vi "CostEvaluation.vi"(0 "Packet Size":i32, 1 "Ratio":dbl format="%#_13g", 3 "Channel":T1, 4 "method":enum16{"Edited", "original"}(ring)) -> (5 "delay(s)":dbl)   [LabVIEW 2014]
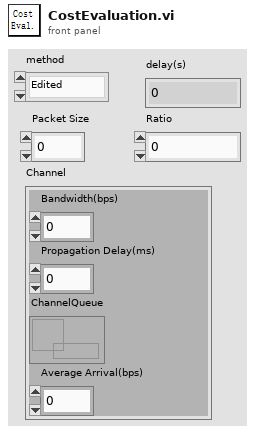
[diagram p1: front panel]
types:
  T1 = cluster{"Bandwidth(bps)":i32, "Propagation Delay(ms)":i32, "ChannelQueue":refnum<queue>, "Average Arrival(bps)":dbl}
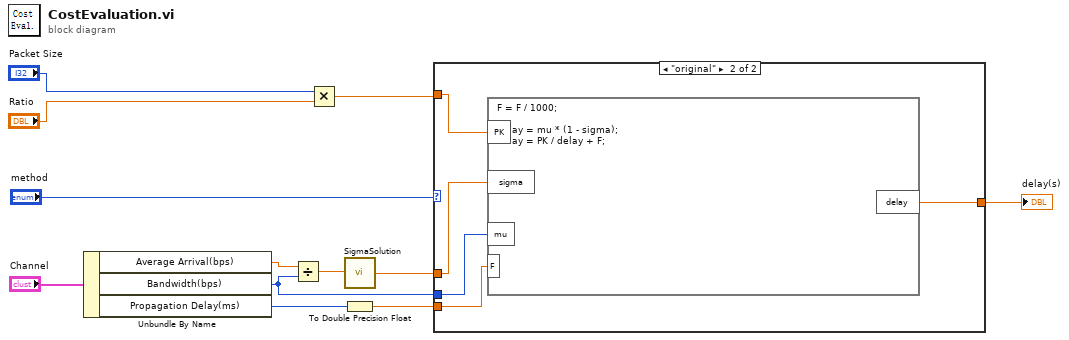
[diagram p0: block diagram]
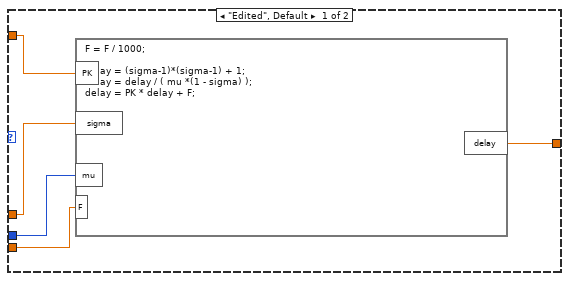
[diagram p2: hidden frame]
diagram:
  n1 = Unbundle By Name("Channel") -> ("Average Arrival(bps)"=w7:dbl, "Bandwidth(bps)"=w3:i32, "Propagation Delay(ms)"=w4:i32)
  n2 = Divide(x=w7, y=w3) -> (x/y=w6:dbl)
  n3 = Multiply(x="Packet Size", y="Ratio") -> (x*y=w9:dbl)
  n4 = call "SigmaSolution.vi"("rou"=w6) -> ("sigma"=w5:dbl)
  n5 = To Double Precision Float(number=w4) -> (double precision float=w1:dbl)
  n6 = case shown="\"original\"" "method" {
    tunnel: w9 -> [w17 w22]
    tunnel: w5 -> [w16 w20]
    tunnel: w1 -> [w14 w18]
    tunnel: w3 -> [w15 w19]
    tunnel: [w13 w21] -> w2
    frame "Edited", Default {
      n7 = formula code="F = F / 1000;\n\ndelay = (sigma-1)*(sigma-1) + 1;\ndelay = delay / ( mu *(1 - sigma) );\ndelay = PK * delay + F;"("PK"=w17, "sigma"=w16, "mu"=w15, "F"=w14) -> ("delay"=w13:dbl)
    }
    frame "original" {
      n8 = formula code="F = F / 1000;\n\ndelay = mu * (1 - sigma);\ndelay = PK / delay + F;"("PK"=w22, "sigma"=w20, "mu"=w19, "F"=w18) -> ("delay"=w21:dbl)
    }
  }
  "delay(s)" <- w2
